vi "READ_SCOPETRACES.vi"() -> ()   [LabVIEW 2013]
panel:
  in  "Export folder":bool
  in  "Export file":bool
  in  "Files":i32[](listbox)=[7]
  out "filenames":string[](array[string])=["TREX PXI slow_026.dat", "TREX PXI slow_027.dat", "TREX PXI slow_028.dat", "TREX PXI slow_029.dat", "TREX PXI slow_030.dat", "TREX PXI slow_031.dat", "TREX PXI slow_032.dat", "TREX PXI slow_033.dat", "TREX PXI slow_034.dat", "TREX PXI slow_035.dat", "TREX PXI slow_036.dat", "TREX PXI slow_037.dat", "TREX PXI slow_038.dat"]
  in  "pattern":string="*.dat"
  in  "Folder path":path=path "W:/USER/Thomas/temp"
  out "number of waveforms":i32=8
  out "ChannelNAmes":string[](array[string])=["0", "1", "2", "3", "4", "5", "6", "7"]
  in  "stop":bool
  in  "Channels":i32[](listbox)=[1]
  in  "file path (dialog if empty)":path=path "W:/USER/Thomas/temp/TREX PXI slow_033.dat"
  out "Waveform Graph":waveform(dbl)[](graph)=[{"t0"=timestamp(0 s since 1904-01-01), "dt"=1.6666666666666667e-08, "Y"=array[100000 elements], "attributes"=variant("Plot.Name"=variant(string "0"))}, {"t0"=timestamp(0 s since 1904-01-01), "dt"=1.6666666666666667e-08, "Y"=array[100000 elements], "attributes"=variant("Plot.Name"=variant(string "1"))}, {"t0"=timestamp(0 s since 1904-01-01), "dt"=1.6666666666666667e-08, "Y"=array[100000 elements], "attributes"=variant("Plot.Name"=variant(string "2"))}, {"t0"=timestamp(0 s since 1904-01-01), "dt"=1.6666666666666667e-08, "Y"=array[100000 elements], "attributes"=variant("Plot.Name"=variant(string "3"))}, {"t0"=timestamp(0 s since 1904-01-01), "dt"=1.6666666666666667e-08, "Y"=array[100000 elements], "attributes"=variant("Plot.Name"=variant(string "4"))}, {"t0"=timestamp(0 s since 1904-01-01), "dt"=1.6666666666666667e-08, "Y"=array[100000 elements], "attributes"=variant("Plot.Name"=variant(string "5"))}, {"t0"=timestamp(0 s since 1904-01-01), "dt"=1.6666666666666667e-08, "Y"=array[100000 elements], "attributes"=variant("Plot.Name"=variant(string "6"))}, {"t0"=timestamp(0 s since 1904-01-01), "dt"=1.6666666666666667e-08, "Y"=array[100000 elements], "attributes"=variant("Plot.Name"=variant(string "7"))}]
  out "error":string
  out "Slide":u8(slide)=1 scale=-1.0..5.0
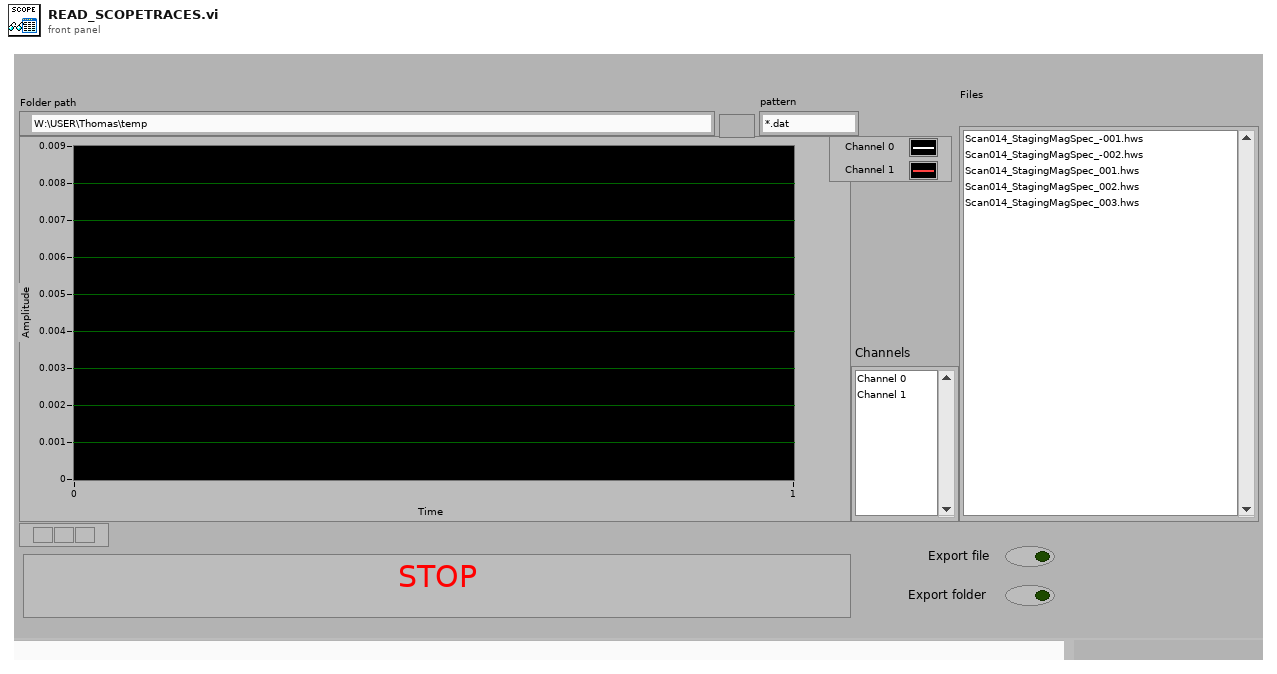
[diagram p1: front panel]
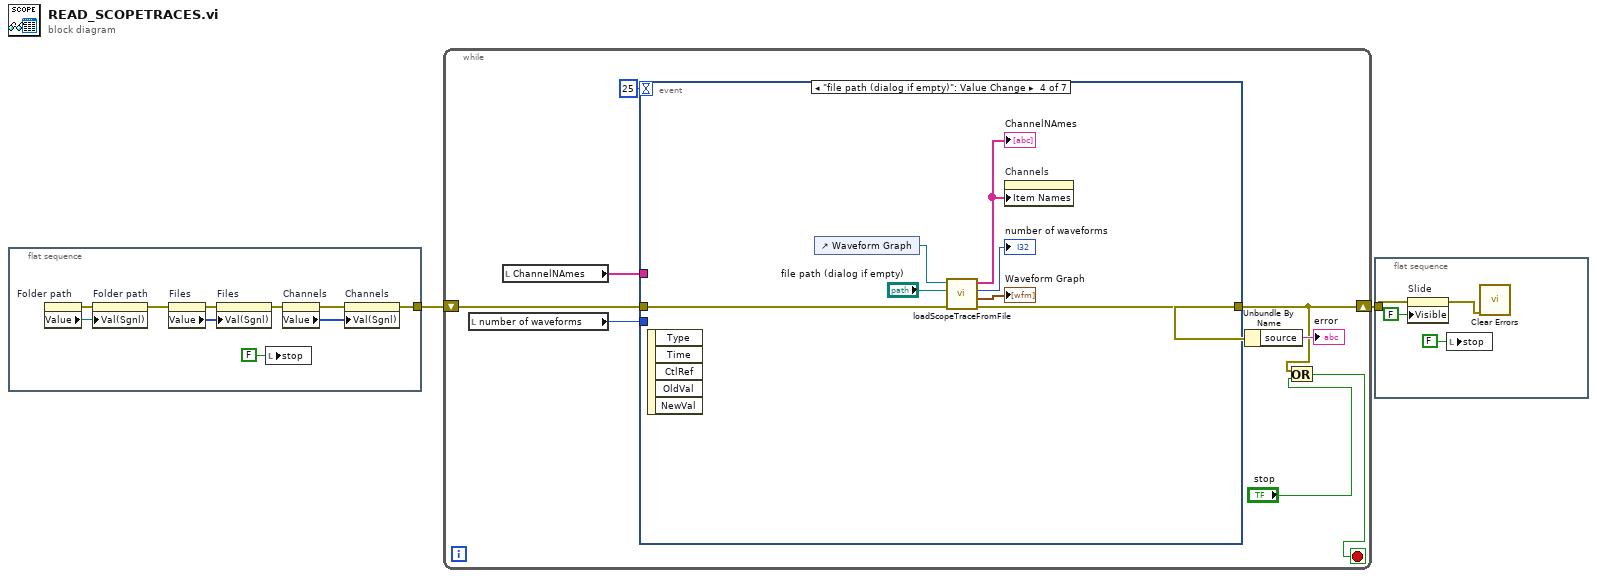
[diagram p0: block diagram]
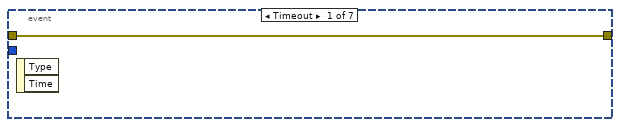
[diagram p2: hidden frame]
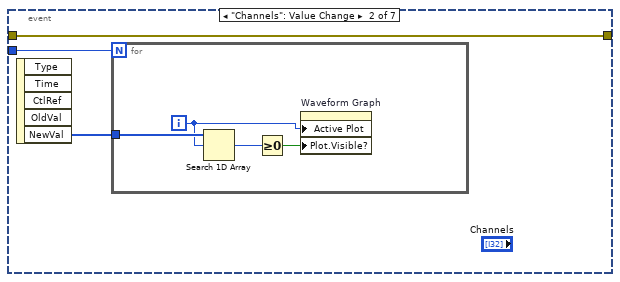
[diagram p3: hidden frame]
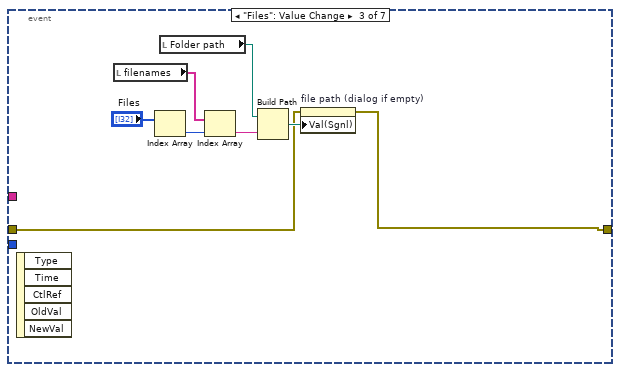
[diagram p4: hidden frame]
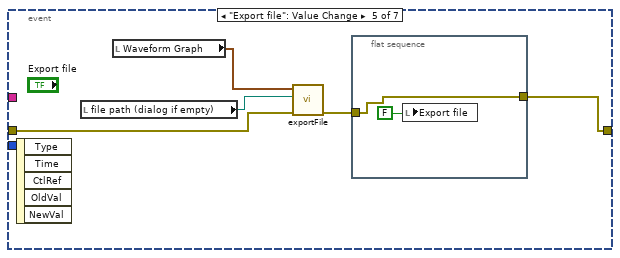
[diagram p5: hidden frame]
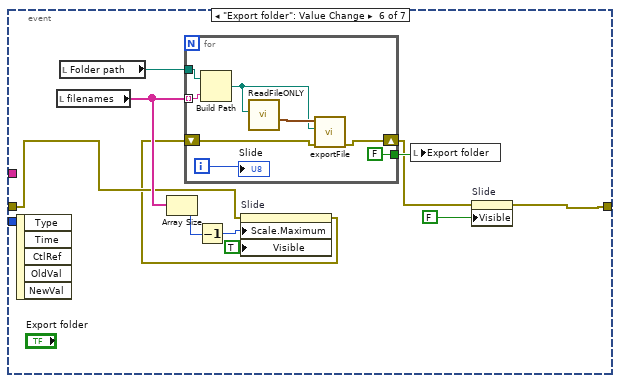
[diagram p6: hidden frame]
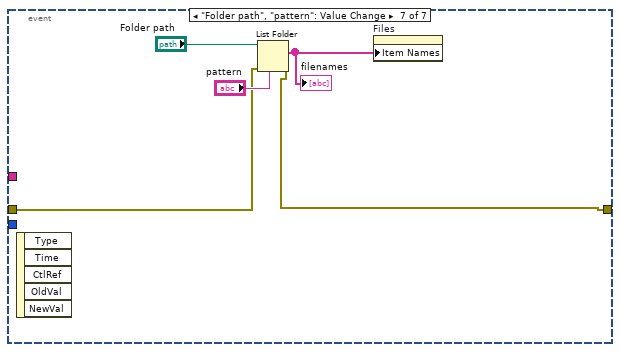
[diagram p7: hidden frame]
diagram:
  n1 = flat-sequence {
    tunnel: [w10] -> w2
    frame #0 {
      n2 = property on="Folder path" class="Path"() -> (error out=w8:errorcluster, "Value"=w9:path)  [unwired: 2 in, 1 out]
      n3 = property on="Folder path" class="Path"(error in=w8, "Val(Sgnl)"=w9) -> (error out=w7:errorcluster)  [unwired: 1 in, 1 out]
      n4 = property on="Files" class="LstBox (strict)"(error in=w7) -> (error out=w6:errorcluster, "Value"=w4:i32[])  [unwired: 1 in, 1 out]
      n5 = property on="Files" class="LstBox (strict)"(error in=w6, "Val(Sgnl)"=w4) -> (error out=w5:errorcluster)  [unwired: 1 in, 1 out]
      n6 = local write "stop"(FALSE ("stop")) -> ()
      n7 = property on="Channels" class="LstBox (strict)"(error in=w5) -> (error out=w11:errorcluster, "Value"=w12:i32[])  [unwired: 1 in, 1 out]
      n8 = property on="Channels" class="LstBox (strict)"(error in=w11, "Val(Sgnl)"=w12) -> (error out=w10:errorcluster)  [unwired: 1 in, 1 out]
    }
  }
  n9 = while {
    shift-right: [w15] -> w1
    shift-left: w2 -> [w17]
    stop <- w13 stop-if-true
    n10 = local read "number of waveforms"() -> (w18:i32)
    n11 = local read "ChannelNAmes"() -> (w19:string[])
    n12 = event shown="[3] \"file path (dialog if empty)\": Value Change" {
      selector: _ -> [_ _ _ _ _ _ _]
      dyn-events: _ -> [_ _ _ _ _ _ _]
      timeout: 25 -> [_ _ _ _ _ _ _]
      tunnel: w19 -> [_ _ _ _ _ _ _]
      tunnel: w18 -> [_ w24 _ _ _ _ _]
      tunnel: [w21 w22 w29 w38 w44 w52 w70] -> w15
      tunnel: w17 -> [w21 w22 w30 w37 w45 w55 w71]
      event Timeout {
        n13 = event-data() -> ()  [unwired: 1 in, 2 out]
      }
      event "Channels": Value Change {
        n14 = event-data() -> ("NewVal"=w23:i32[])  [unwired: 1 in, 4 out]
        n15 = for {
          N: w24 -> [_]
          tunnel: w23 -> [w28]
          i -> [w27]
          n16 = Search 1D Array(1D array=w28, element=w27) -> (index of element=w26:i32)  [unwired: 1 in]
          n17 = Greater Or Equal To 0?(x=w26) -> (x >= 0?=w25:bool)
          n18 = property on="Waveform Graph" class="WFGraph (strict)"("Active Plot"=w27, "Plot.Visible?"=w25) -> ()  [unwired: 2 in, 2 out]
        }
      }
      event "Files": Value Change {
        n19 = event-data() -> ()  [unwired: 1 in, 5 out]
        n20 = local read "filenames"() -> (w36:string[])
        n21 = Index Array(array="Files") -> (element=w34:i32)  [unwired: 1 in]
        n22 = local read "Folder path"() -> (w33:path)
        n23 = Index Array(array=w36, index=w34) -> (element=w32:string)
        n24 = Build Path(base path=w33, name or relative path=w32) -> (appended path=w31:path)
        n25 = property on="file path (dialog if empty)" class="Path"(error in=w30, "Val(Sgnl)"=w31) -> (error out=w29:errorcluster)  [unwired: 1 in, 1 out]
      }
      event "file path (dialog if empty)": Value Change {
        n26 = event-data() -> ()  [unwired: 1 in, 5 out]
        n27 = control-ref of="Waveform Graph"() -> (w43:refnum<vi>)
        n28 = call "loadScopeTraceFromFile.vi"("error in (no error)"=w37, "file path (dialog if empty)"="file path (dialog if empty)", "WaveformGraph in"=w43) -> ("error out"=w38:errorcluster, "Array 2"=→"Waveform Graph":waveform(dbl)[], "number of waveforms"=→"number of waveforms":i32, "Array"=w41:string[])  [unwired: 5 in]
        "ChannelNAmes" <- w41
        n29 = property on="Channels" class="LstBox (strict)"("Item Names"=w41) -> ()  [unwired: 2 in, 2 out]
      }
      event "Export file": Value Change {
        n30 = event-data() -> ()  [unwired: 1 in, 5 out]
        n31 = local read "file path (dialog if empty)"() -> (w47:path)
        n32 = local read "Waveform Graph"() -> (w48:waveform(dbl)[])
        n33 = call "exportFile.vi"("error in"=w45, "file path (dialog if empty)"=w47, "Waveform Graph"=w48) -> ("error out"=w46:errorcluster)  [unwired: 8 in]
        n34 = flat-sequence {
          tunnel: w46 -> [w49]
          tunnel: [w49] -> w44
          frame #0 {
            n35 = local write "Export file"(FALSE) -> ()
          }
        }
      }
      event "Export folder": Value Change {
        n36 = event-data() -> ()  [unwired: 1 in, 5 out]
        n37 = local read "filenames"() -> (w59:string[])
        n38 = local read "Folder path"() -> (w61:path)
        n39 = Array Size(array=w59) -> (size(s)=w58:i32)
        n40 = Decrement(x=w58) -> (x-1=w57:i32)
        n41 = property on="Slide" class="Slide (strict)"(error in=w55, "Scale.Maximum"=w57, "Visible"=TRUE) -> (error out=w54:errorcluster)  [unwired: 1 in, 1 out]
        n42 = for {
          tunnel: w59 -> [w68] mode=indexing
          tunnel: w61 -> [w67]
          tunnel: [FALSE] -> w60
          shift-right: [w64] -> w53
          shift-left: w54 -> [w65]
          i -> [w62]
          n43 = Build Path(base path=w67, name or relative path=w68) -> (appended path=w63:path)
          n44 = call "ReadFileONLY.vi"("file path (dialog if empty)"=w63) -> ("Waveform Graph"=w69:waveform(dbl)[])  [unwired: 5 in, 5 out]
          n45 = call "exportFile.vi"("error in"=w65, "file path (dialog if empty)"=w63, "Waveform Graph"=w69) -> ("error out"=w64:errorcluster)  [unwired: 8 in]
          "Slide" <- w62
        }
        n46 = local write "Export folder"(w60) -> ()
        n47 = property on="Slide" class="Slide (strict)"(error in=w53, "Visible"=FALSE) -> (error out=w52:errorcluster)  [unwired: 1 in, 1 out]
      }
      event "Folder path", "pattern": Value Change {
        n48 = event-data() -> ()  [unwired: 1 in, 5 out]
        n49 = List Folder(path="Folder path", pattern="pattern", error in=w71) -> (filenames=w74:string[], error out=w70:errorcluster)  [unwired: 1 in, 2 out]
        "filenames" <- w74
        n50 = property on="Files" class="LstBox (strict)"("Item Names"=w74) -> ()  [unwired: 2 in, 2 out]
      }
    }
    n51 = Unbundle By Name(w15) -> ("source"=→"error":string)
    n52 = Or(x=w15, y="stop") -> (x .or. y?=w13:bool)
  }
  n53 = flat-sequence {
    tunnel: w1 -> [w78]
    frame #0 {
      n54 = property on="Slide" class="Slide (strict)"(error in=w78, "Visible"=FALSE) -> (error out=w75:errorcluster)  [unwired: 1 in, 1 out]
      n55 = local write "stop"(FALSE ("stop")) -> ()
      n56 = call <vilib>:"Clear Errors.vi"("error in (no error)"=w75) -> ()  [unwired: 6 in, 1 out]
    }
  }
